vi "数据处理整合 (子VI).vi"(11 "枚举":enum16{"实时数据排序", "小时数据排序"}(ring)) -> (3 "已排序的数组":string[](array[string]))   [LabVIEW 2016, in "数据传输系统.lvlib"]
uses:
  <userlib>/_OpenG.lib/array/array.llb/Remove Duplicates from 1D Array (String)__ogtk.vi
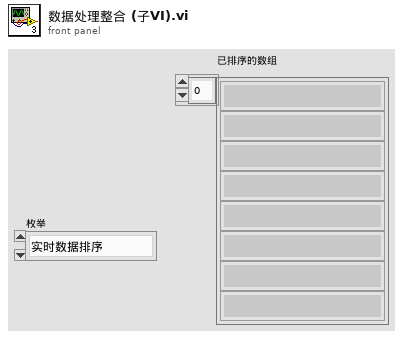
[diagram p1: front panel]
types:
  T1 = cluster{"PH":string[][], "CODCr":string[][], "氨氮":string[][], "CODMn":string[][], "总氮":string[][], "总磷":string[][], "电导率":string[][], "水温":string[][], "DO":string[][], "浊度":string[][], "叶绿素":string[][], "藻密度":string[][], "铜":string[][], "盐度":string[][], "水位":string[][], "流速":string[][], "瞬时流量":string[][], "累积流量":string[][]}
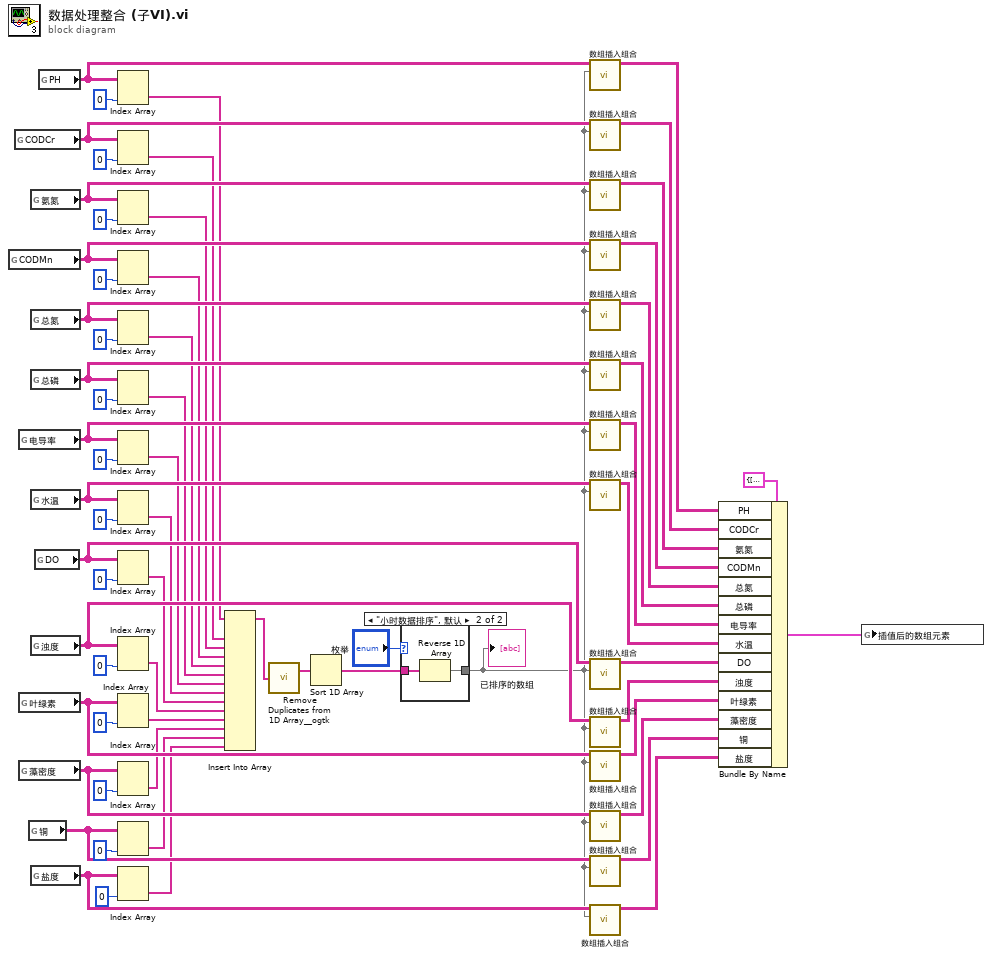
[diagram p0: block diagram]
diagram:
  n1 = global read "全局 所有参数.vi" "CODMn"() -> (w44:string[][])
  n2 = global read "全局 所有参数.vi" "CODCr"() -> (w42:string[][])
  n3 = global read "全局 所有参数.vi" "电导率"() -> (w47:string[][])
  n4 = global read "全局 所有参数.vi" "叶绿素"() -> (w51:string[][])
  n5 = global read "全局 所有参数.vi" "藻密度"() -> (w52:string[][])
  n6 = global read "全局 所有参数.vi" "铜"() -> (w11:string[][])
  n7 = global read "全局 所有参数.vi" "氨氮"() -> (w43:string[][])
  n8 = global read "全局 所有参数.vi" "总氮"() -> (w45:string[][])
  n9 = global read "全局 所有参数.vi" "总磷"() -> (w46:string[][])
  n10 = global read "全局 所有参数.vi" "水温"() -> (w48:string[][])
  n11 = global read "全局 所有参数.vi" "浊度"() -> (w50:string[][])
  n12 = global read "全局 所有参数.vi" "盐度"() -> (w10:string[][])
  n13 = global read "全局 所有参数.vi" "DO"() -> (w49:string[][])
  n14 = global read "全局 所有参数.vi" "PH"() -> (w40:string[][])
  n15 = Index Array(array=w40, index (col)=0 ("索引 (行)")) -> (element=w27:string[])  [unwired: 1 in]
  n16 = Index Array(array=w42, index (col)=0 ("索引 (行)")) -> (element=w28:string[])  [unwired: 1 in]
  n17 = Index Array(array=w43, index (col)=0 ("索引 (行)")) -> (element=w29:string[])  [unwired: 1 in]
  n18 = Index Array(array=w44, index (col)=0 ("索引 (行)")) -> (element=w30:string[])  [unwired: 1 in]
  n19 = Index Array(array=w45, index (col)=0 ("索引 (行)")) -> (element=w31:string[])  [unwired: 1 in]
  n20 = Index Array(array=w46, index (col)=0 ("索引 (行)")) -> (element=w32:string[])  [unwired: 1 in]
  n21 = Index Array(array=w47, index (col)=0 ("索引 (行)")) -> (element=w33:string[])  [unwired: 1 in]
  n22 = Index Array(array=w48, index (col)=0 ("索引 (行)")) -> (element=w34:string[])  [unwired: 1 in]
  n23 = Index Array(array=w49, index (col)=0 ("索引 (行)")) -> (element=w35:string[])  [unwired: 1 in]
  n24 = Index Array(array=w50, index (col)=0 ("索引 (行)")) -> (element=w36:string[])  [unwired: 1 in]
  n25 = Index Array(array=w51, index (col)=0 ("索引 (行)")) -> (element=w37:string[])  [unwired: 1 in]
  n26 = Index Array(array=w52, index (col)=0 ("索引 (行)")) -> (element=w38:string[])  [unwired: 1 in]
  n27 = Index Array(array=w11, index (col)=0 ("索引 (行)")) -> (element=w9:string[])  [unwired: 1 in]
  n28 = Index Array(array=w10, index (col)=0 ("索引 (行)")) -> (element=w8:string[])  [unwired: 1 in]
  n29 = Insert Into Array(array=w27, new element #1=w28, new element #2=w29, new element #3=w30, new element #4=w31, new element #5=w32, new element #6=w33, new element #7=w34, new element #8=w35, new element #9=w36, new element #10=w37, new element #11=w38, new element #12=w9, new element #13=w8) -> (w39:string[])  [unwired: 1 in]
  n30 = call-poly <userlib>:"Remove Duplicates from 1D Array__ogtk.vi"("Input Array"=w39) -> ("Output Array"=w26:string[])  [unwired: 1 out]
  n31 = Sort 1D Array(array=w26) -> (sorted array=w12:string[])
  n32 = case shown="\"小时数据排序\", 默认" "枚举" {
    tunnel: w12 -> [w64 w66]
    tunnel: [w64 w65] -> w7
    frame "实时数据排序" {
    }
    frame "小时数据排序", Default {
      n33 = Reverse 1D Array(array=w66) -> (reversed array=w65:string[])
    }
  }
  "已排序的数组" <- w7
  n34 = call "数组插入组合.vi"("排序后的一维数组"=w7, "输入数组"=w40) -> ("输出结果"=w41:string[][])  [unwired: 9 in]
  n35 = call "数组插入组合.vi"("排序后的一维数组"=w7, "输入数组"=w42) -> ("输出结果"=w53:string[][])  [unwired: 9 in]
  n36 = call "数组插入组合.vi"("排序后的一维数组"=w7, "输入数组"=w43) -> ("输出结果"=w54:string[][])  [unwired: 9 in]
  n37 = call "数组插入组合.vi"("排序后的一维数组"=w7, "输入数组"=w44) -> ("输出结果"=w55:string[][])  [unwired: 9 in]
  n38 = call "数组插入组合.vi"("排序后的一维数组"=w7, "输入数组"=w45) -> ("输出结果"=w56:string[][])  [unwired: 9 in]
  n39 = call "数组插入组合.vi"("排序后的一维数组"=w7, "输入数组"=w46) -> ("输出结果"=w57:string[][])  [unwired: 9 in]
  n40 = call "数组插入组合.vi"("排序后的一维数组"=w7, "输入数组"=w47) -> ("输出结果"=w58:string[][])  [unwired: 9 in]
  n41 = call "数组插入组合.vi"("排序后的一维数组"=w7, "输入数组"=w48) -> ("输出结果"=w59:string[][])  [unwired: 9 in]
  n42 = call "数组插入组合.vi"("排序后的一维数组"=w7, "输入数组"=w49) -> ("输出结果"=w60:string[][])  [unwired: 9 in]
  n43 = call "数组插入组合.vi"("排序后的一维数组"=w7, "输入数组"=w50) -> ("输出结果"=w61:string[][])  [unwired: 9 in]
  n44 = call "数组插入组合.vi"("排序后的一维数组"=w7, "输入数组"=w51) -> ("输出结果"=w62:string[][])  [unwired: 9 in]
  n45 = call "数组插入组合.vi"("排序后的一维数组"=w7, "输入数组"=w52) -> ("输出结果"=w63:string[][])  [unwired: 9 in]
  n46 = call "数组插入组合.vi"("排序后的一维数组"=w7, "输入数组"=w11) -> ("输出结果"=w6:string[][])  [unwired: 9 in]
  n47 = call "数组插入组合.vi"("排序后的一维数组"=w7, "输入数组"=w10) -> ("输出结果"=w5:string[][])  [unwired: 9 in]
  n48 = Bundle By Name(cluster=T1 {"PH"=[], "CODCr"=[], "氨氮"=[], "CODMn"=[], "总氮"=[], "总磷"=[], "电导率"=[], "水温"=[], "DO"=[], "浊度"=[], "叶绿素"=[], "藻密度"=[], "铜"=[], "盐度"=[], "水位"=[], "流速"=[], "瞬时流量"=[], "累积流量"=[]} ("插值后的数组元素"), "PH"=w41, "CODCr"=w53, "氨氮"=w54, "CODMn"=w55, "总氮"=w56, "总磷"=w57, "电导率"=w58, "水温"=w59, "DO"=w60, "浊度"=w61, "叶绿素"=w62, "藻密度"=w63, "铜"=w6, "盐度"=w5) -> (w1:T1)
  n49 = global write "插值后的新数组.vi" "插值后的数组元素"(w1) -> ()
